vi "ant_in_home.vi"(1 "pieceOfWorld":T1[][](array[typedef])) -> (0 "x .and. y?":bool)   [LabVIEW 2015, in "PolyVIEW.lvclass"]
uses:
  PolyVIEW.lvclass
  actors/world/typedefs/worldCell_cluster.ctl
  actors/world/typedefs/markValue_cluster.ctl
  actors/world/typedefs/markValue.ctl
  actors/world/typedefs/markVolume.ctl
  actors/world/typedefs/amountOfFood.ctl
  actors/world/typedefs/anthillType_enum.ctl
  actors/world/world.lvlib
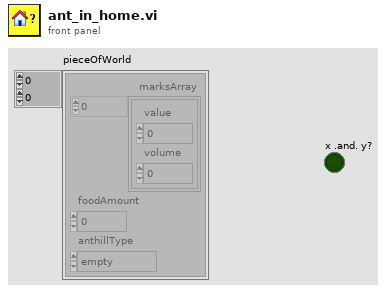
[diagram p1: front panel]
types:
  T1 = typedef "world.lvlib/worldCell_cluster.ctl" = cluster{"marksArray":T2[], "foodAmount":T5, "anthillType":T6}
  T2 = typedef "world.lvlib/markValue_cluster.ctl" = cluster{"value":T3, "volume":T4}
  T3 = typedef "world.lvlib/markValue.ctl" = u8
  T4 = typedef "world.lvlib/markVolume.ctl" = u16
  T5 = typedef "world.lvlib/amountOfFood.ctl" = i32
  T6 = typedef "world.lvlib/anthillType_enum.ctl" = enum16{"empty", "own", "rival"}
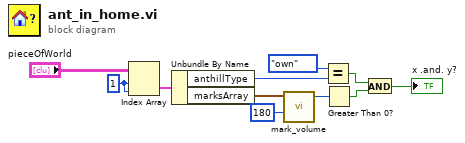
[diagram p0: block diagram]
diagram:
  w5 = 1 ("index (row)")
  n1 = Index Array(array="pieceOfWorld", index (row)=w5, index (col)=w5) -> (element=w4:T1)
  n2 = Unbundle By Name(w4) -> ("anthillType"=w2:T6, "marksArray"=w3:T2[])
  n3 = call "mark_volume.vi"("element"=T3 180, "marksArray"=w3) -> ("volume"=w8:T4)  [unwired: 9 in]
  n4 = Equal?(x=anthillType_enum."own" ("y"), y=w2) -> (x = y?=w10:bool)
  n5 = Greater Than 0?(x=w8) -> (x > 0?=w7:bool)
  n6 = And(x=w10, y=w7) -> (x .and. y?=→"x .and. y?":bool)
